vi "File_I:O(Binary).vi"() -> ()   [LabVIEW 2023]
panel:
  out "data 2":dbl[](graph)
  out "data":dbl[](array[numeric])
  in  "file path (use dialog) 2":path
  in  "file path (use dialog)":path
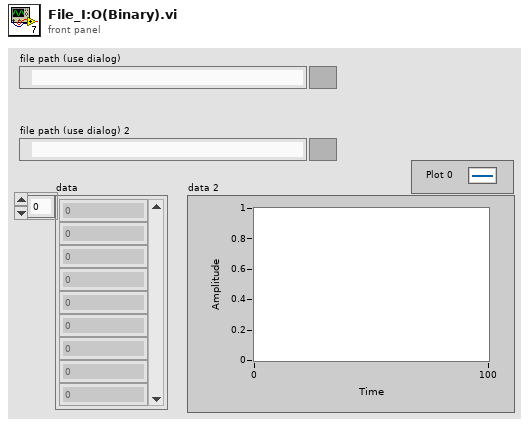
[diagram p1: front panel]
types:
  T1 = enum16{"open", "replace", "create", "open or create", "replace or create", "replace or create with confirmation"}
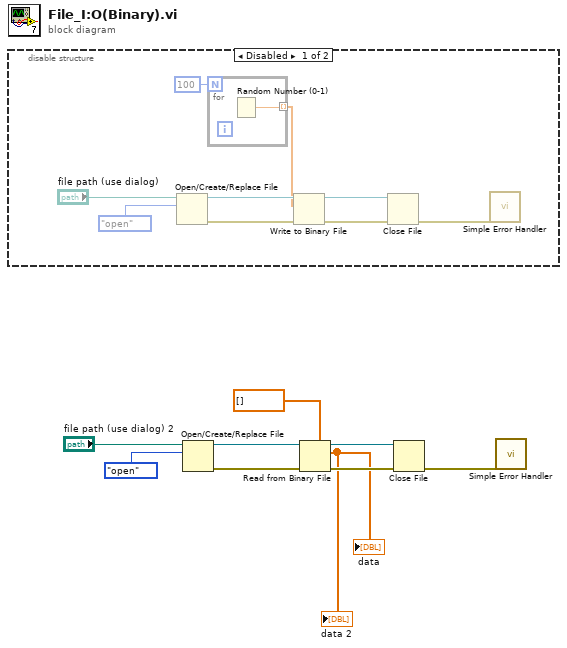
[diagram p0: block diagram]
diagram:
  n1 = disable-structure shown="Disabled" {
    frame Disabled {
      n2 = Open/Create/Replace File(file path (use dialog)="file path (use dialog)", operation (0:open)=T1."open") -> (refnum out=w16:refnum<file>, error out=w14:errorcluster)  [unwired: 4 in, 1 out]
      n3 = for {
        N: 100 -> [_]
        tunnel: [w19] -> w10 mode=indexing
        n4 = Random Number (0-1)() -> (number: 0 to 1=w19:dbl)
      }
      n5 = Write to Binary File(file (use dialog)=w16, data=w10, error in=w14) -> (refnum out=w15:refnum<file>, error out=w13:errorcluster)  [unwired: 3 in, 1 out]
      n6 = Close File(refnum=w15, error in=w13) -> (error out=w12:errorcluster)  [unwired: 1 out]
      n7 = call <vilib>:"Simple Error Handler.vi"("error in (no error)"=w12) -> ()  [unwired: 4 in, 5 out]
    }
    frame Enabled {
    }
  }
  n8 = Open/Create/Replace File(file path (use dialog)="file path (use dialog) 2", operation (0:open)=T1."open") -> (refnum out=w7:refnum<file>, error out=w5:errorcluster)  [unwired: 4 in, 1 out]
  n9 = Read from Binary File(5:dbl[] [], 8:w5, 11:w7) -> (0:w4:errorcluster, 2:→"data" →"data 2":dbl[], 3:w6:refnum<file>)  [unwired: 3 in, 1 out]
  n10 = Close File(refnum=w6, error in=w4) -> (error out=w3:errorcluster)  [unwired: 1 out]
  n11 = call <vilib>:"Simple Error Handler.vi"("error in (no error)"=w3) -> ()  [unwired: 4 in, 5 out]
